vi "GenerateChangedFilesList.vi"(6 "GUI Mode? {F)":bool, 8 "error in (no error)":errorcluster) -> (0 "error out":errorcluster)   [LabVIEW 2023, in "CheckModifiedVIs.lvlib"]
uses:
  CheckModifiedVIs.lvlib
  <vilib>/Hampel Software Engineering/Git API/Git API/GIT-api.lvclass/GIT-api.ctl
  <vilib>/Hampel Software Engineering/Git API/Git API/Accessors/GIT-Set Working Dir.vi
  <vilib>/Wiresmith Technology/G CLI/CLI Class/CLI.lvclass
  <vilib>/Hampel Software Engineering/Git API/Git API/GIT-api.lvclass
  Reusables/Reusables.lvlib
panel:
  out "std out":string
  in  "Tab Control":T1(tab)
  in  "Output File Path":path=path "E:/sw-deps-monitor/changed-files.txt"
  in  "Branch 2":string="initial-ci-check-yml"
  in  "Branch 1":string="main"
  in  "Workspace Path":path=path "E:/sw-deps-monitor"
  out "Args":string[](array[string])=["E:\\sw-deps-monitor", "main", "initial-ci-check-yml", "E:\\sw-deps-monitor\\changed-files.txt"]
  # "When in GUI Mode, the controls will be used, \nin CLI Mode the Args will be used"
  # "Workspace Path"
  # "Branch 1"
  # "Branch 2"
  # "Output File Path"
  # "Command to run the VI from terminal\n\ng-cli -v --lv-ver 2023 --arch 32 \"E:\\sw-deps-monitor\\CICD\\Reusables\\GenerateChangedFilesList.vi\" \n-- \"E:\\sw-deps-monitor\" \"main\" \"initial-ci-check-yml\" \"E:\\sw-deps-monitor\\changed-files.txt\""
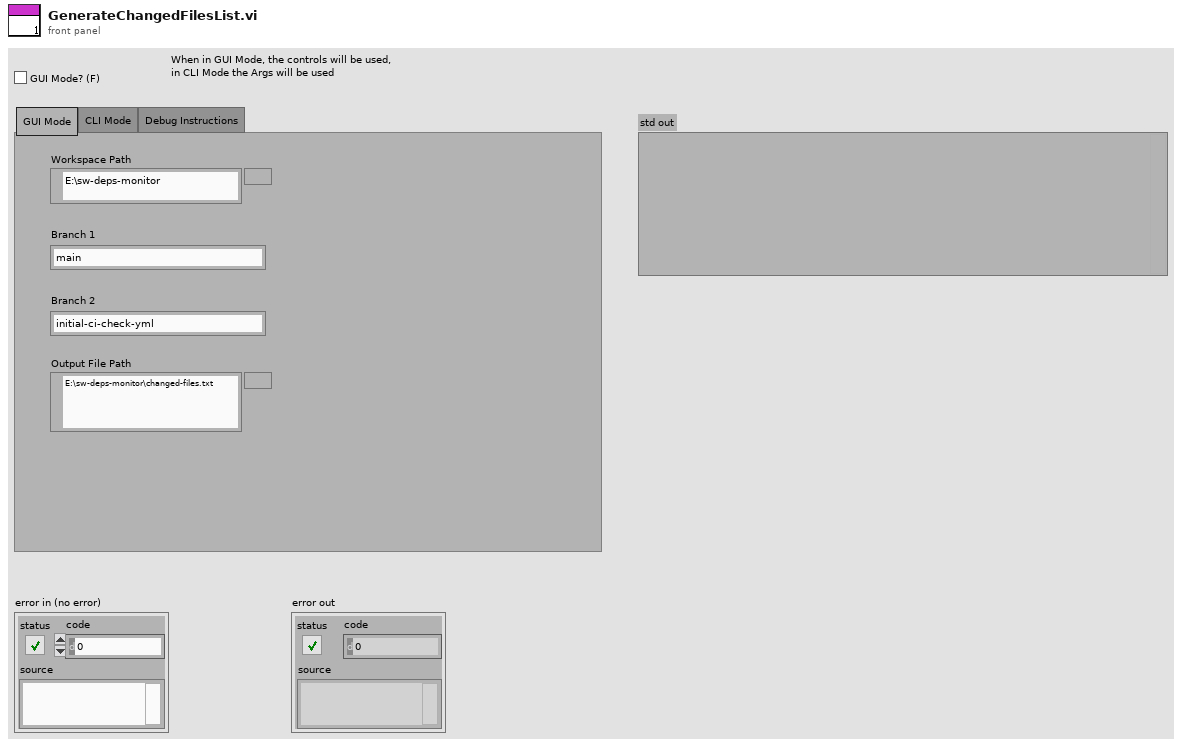
[diagram p1: front panel]
types:
  T1 = enum32{"GUI Mode", "CLI Mode", "Debug Instructions"}
  T2 = enum16{"open", "replace", "create", "open or create", "replace or create", "replace or create with confirmation"}
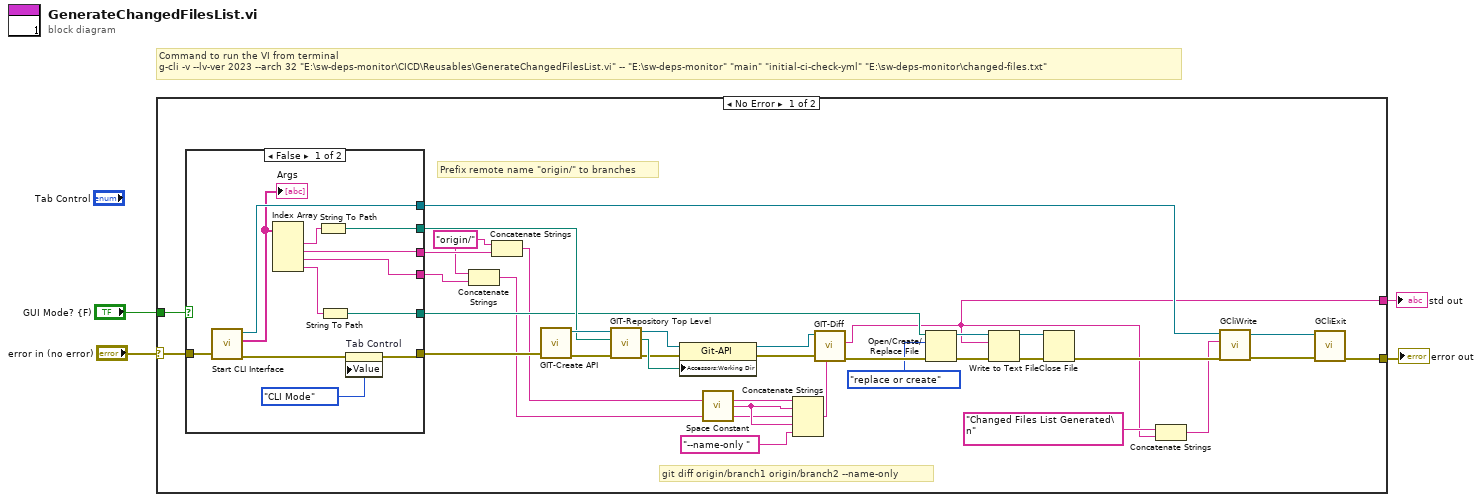
[diagram p0: block diagram]
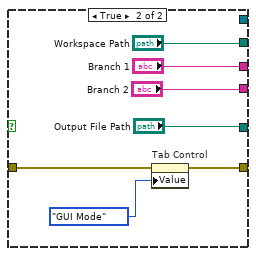
[diagram p2: hidden frame]
diagram:
  # "Command to run the VI from terminal\ng-cli -v --lv-ver 2023 --arch 32 \"E:\\sw-deps-monitor\\CICD\\Reusables\\GenerateChangedFilesList.vi\" -- \"E:\\sw-deps-monitor\" \"main\" \"initial-ci-check-yml\" \"E:\\sw-deps-monitor\\changed-files.txt\""
  n1 = case shown="No Error" "error in (no error)" {
    selector: "error in (no error)" -> [w28 w58]
    tunnel: "GUI Mode? {F)" -> [w29 _]
    tunnel: [w11 _] -> w2
    tunnel: [w14 w58] -> w1
    frame No Error {
      w7 = "origin/" ("string")
      # "git diff origin/branch1 origin/branch2 --name-only"
      # "Prefix remote name \"origin/\" to branches"
      n2 = case shown="False" w29 {
        tunnel: [w49 "Branch 1"] -> w9
        tunnel: [w46 "Workspace Path"] -> w26
        tunnel: [w45 "Output File Path"] -> w23
        tunnel: [w48 "Branch 2"] -> w6
        tunnel: w28 -> [w44 w53]
        tunnel: [w42 w51] -> w27
        tunnel: [w43 _] -> w16
        frame False {
          n3 = call <vilib>:"Start CLI Interface.vi"("error in (no error)"=w44) -> ("error out"=w40:errorcluster, "Custom Parameters"=w39:string[], "CLI out"=w43:refnum<class "CLI.lvclass">)  [unwired: 7 in, 1 out]
          "Args" <- w39
          n4 = Index Array(array=w39) -> (element #1=w50:string, element #2=w49:string, element #3=w48:string, element #4=w47:string)  [unwired: 4 in]
          n5 = String To Path(string=w50) -> (path=w46:path)
          n6 = String To Path(string=w47) -> (path=w45:path)
          n7 = property on="Tab Control" class="TabCtl (strict)"(error in=w40, "Value"=enum32{"GUI Mode", "CLI Mode"}."CLI Mode" ("Tab Control")) -> (error out=w42:errorcluster)  [unwired: 1 in, 1 out]
        }
        frame True {
          n8 = property on="Tab Control" class="TabCtl (strict)"(error in=w53, "Value"=enum32{"GUI Mode", "CLI Mode"}."GUI Mode" ("Tab Control")) -> (error out=w51:errorcluster)  [unwired: 1 in, 1 out]
        }
      }
      n9 = Concatenate Strings(w7, w6) -> (w5:string)
      n10 = Concatenate Strings(w7, w9) -> (w8:string)
      n11 = call <vilib>:"GIT-Create API.vi"("error in"=w27) -> ("error out"=w34:errorcluster, "git-api out"=w37:refnum<class "GIT-api.lvclass">)  [unwired: 9 in]
      n12 = call <vilib>:"GIT-Repository Top Level.vi"("error in"=w34, "Current Path"=w26, "git-api in"=w37) -> ("error out"=w35:errorcluster, "Repo Top Level Path"=w36:path, "git-api out"=w38:refnum<class "GIT-api.lvclass">)  [unwired: 6 in]
      n13 = property class="Git-API"(reference=w38, error in=w35, "Accessors:Working Dir"=w36) -> (reference out=w32:refnum<class "GIT-api.lvclass">, error out=w33:errorcluster)
      n14 = call <vilib>:"Space Constant.vi"() -> ("String"=w25:string)
      n15 = Concatenate Strings(w8, w25, w5, w25, "--name-only " ("string")) -> (w31:string)
      n16 = call <vilib>:"GIT-Diff.vi"("param"=w31, "error in"=w33, "git-api in"=w32) -> ("error out"=w24:errorcluster, "std out"=w11:string)  [unwired: 6 in, 1 out]
      n17 = Open/Create/Replace File(file path (use dialog)=w23, error in=w24, operation (0:open)=T2."replace or create") -> (refnum out=w20:refnum<file>, error out=w21:errorcluster)  [unwired: 3 in, 1 out]
      n18 = Write to Text File(file (use dialog)=w20, text=w11, error in=w21) -> (refnum out=w18:refnum<file>, error out=w19:errorcluster)  [unwired: 1 in, 1 out]
      n19 = Close File(refnum=w18, error in=w19) -> (error out=w17:errorcluster)  [unwired: 1 out]
      n20 = Concatenate Strings("Changed Files List Generated\n" ("Text to Write"), w11) -> (w10:string)
      n21 = call "GCliWrite.vi"("error in (no error)"=w17, "Text to Write"=w10, "CLI in"=w16) -> ("error out"=w15:errorcluster, "CLI out"=w13:refnum<class "CLI.lvclass">)  [unwired: 7 in]
      n22 = call "GCliExit.vi"("error in (no error)"=w15, "CLI in"=w13) -> ("error out"=w14:errorcluster)  [unwired: 9 in]
    }
    frame Error {
    }
  }
  "error out" <- w1
  "std out" <- w2
